vi "Data Display.vi"(8 "error in (no error)":errorcluster, 9 "UI Data Display Cluster":T3, 10 "Message Queues in":T1, 11 "Estimate Notifier in":refnum<notifier>) -> (0 "error out":errorcluster)   [LabVIEW 2019]
uses:
  controls/UI Display.ctl
  <vilib>/Math Plots/2D Math Plots/2D Compass/2D Compass XCtrl/2D Compass.xctl
  support/Message Queue/All Message Queues.ctl
  support/Message Queue/Message Cluster.ctl
  controls/Components Message Queues.ctl
  Data Analysis/EstimateCluster.ctl
  controls/Component Type.ctl
  support/Message Queue/Enqueue Message (Single).vi
  <vilib>/Math Plots/2D Math Plots/2D Compass/2D Compass Datatype/Public/Plot Helper (Vector).vi
  <vilib>/Utility/file.llb/Read Delimited Spreadsheet (DBL).vi
  <vilib>/Math Plots/2D Math Plots/2D Compass/2D Compass Datatype/Public/Plot Helper (Complex).vi
  <vilib>/Utility/error.llb/Error Cluster From Error Code.vi
  <vilib>/ErrorRing/Error Ring.xnode
  support/Message Queue/Message Queue.lvlib
  <vilib>/Math Plots/2D Math Plots/2D Compass/2D Compass Datatype/2D Compass Datatype.lvclass
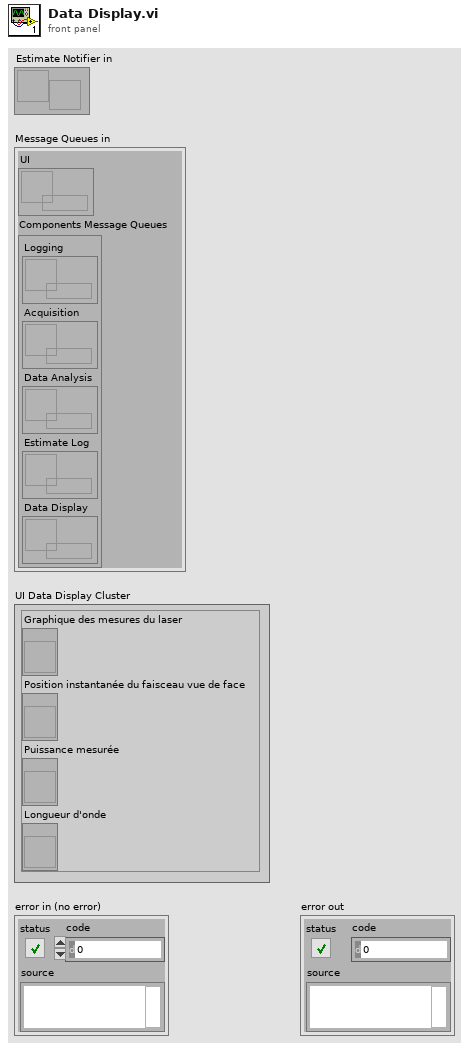
[diagram p1: front panel]
types:
  T1 = typedef "Message Queue.lvlib/All Message Queues.ctl" = cluster{"UI":refnum<queue>, "Components Message Queues":T2}
  T2 = typedef "Message Queue.lvlib/Components Message Queues.ctl" = cluster{"Logging":refnum<queue>, "Acquisition":refnum<queue>, "Data Analysis":refnum<queue>, "Estimate Log":refnum<queue>, "Data Display":refnum<queue>}
  T3 = typedef "UI Display.ctl" = cluster{"Graphique des mesures du laser":refnum<vi>, "Position instantanée du faisceau vue de face":refnum<vi>, "Puissance mesurée":refnum<vi>, "Longueur d'onde":refnum<vi>}
  T4 = typedef "Component Type.ctl" = enum16{"UI", "Logging", "Acquisition", "Data Analysis", "Estimate", "Data Display"}
  T5 = cluster{"all rows[0]":dbl, "all rows[1]":dbl, "all rows[2]":dbl, "all rows[3]":dbl, "all rows[4]":dbl, "all rows[5]":dbl, "all rows[6]":dbl, "all rows[7]":dbl, "all rows[8]":dbl}
  T6 = typedef "EstimateCluster.ctl" = cluster{"Lambda":dbl, "Puissance":dbl, "Rayon":dbl, "Angle":dbl, "dt":dbl, "t0":timestamp}
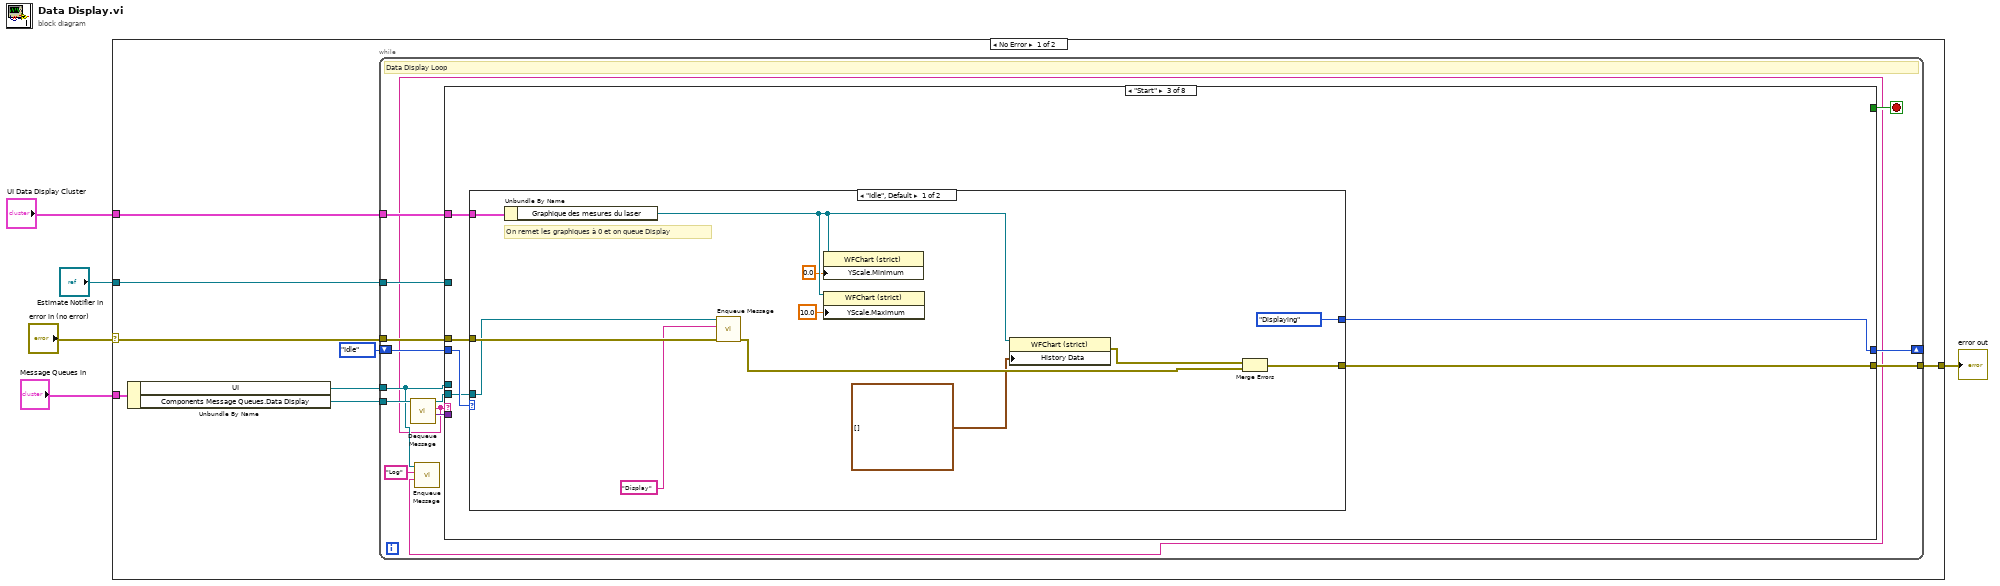
[diagram p0: block diagram]
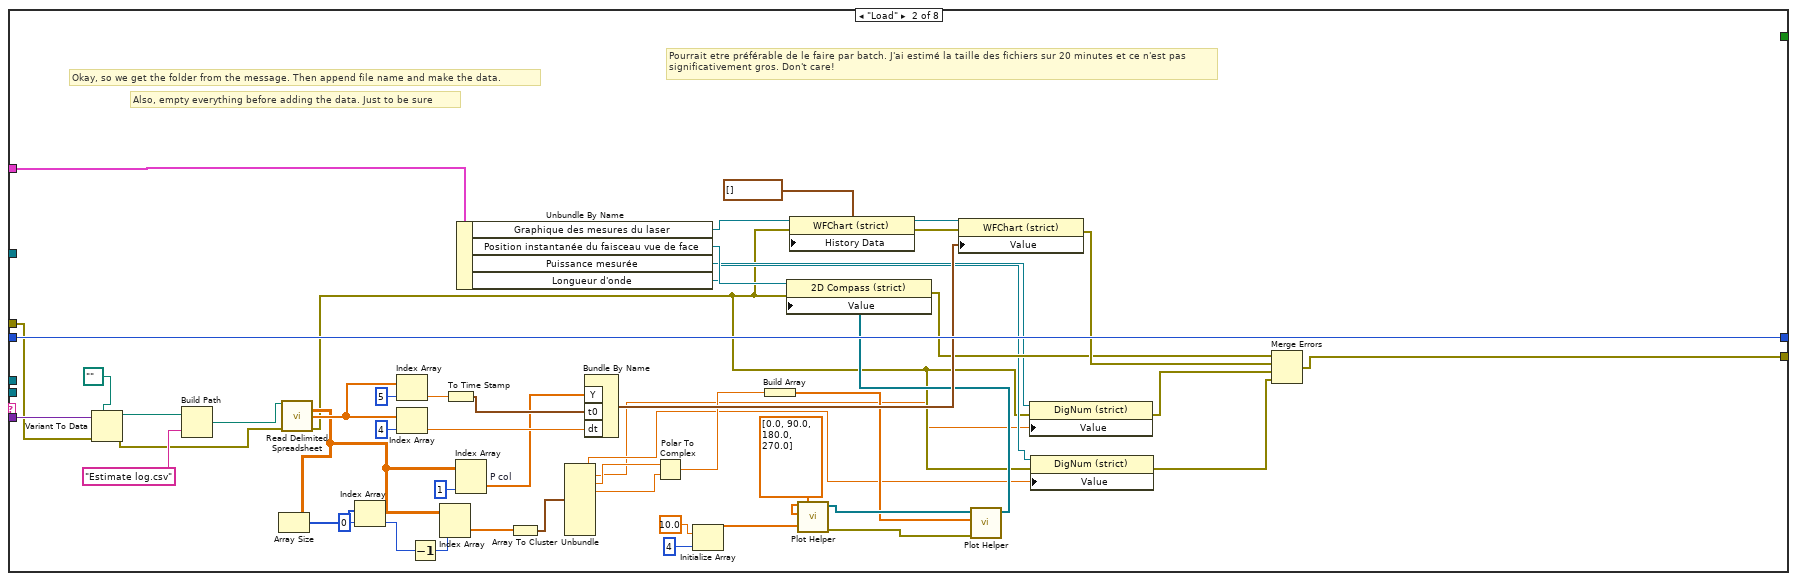
[diagram p3: hidden frame]
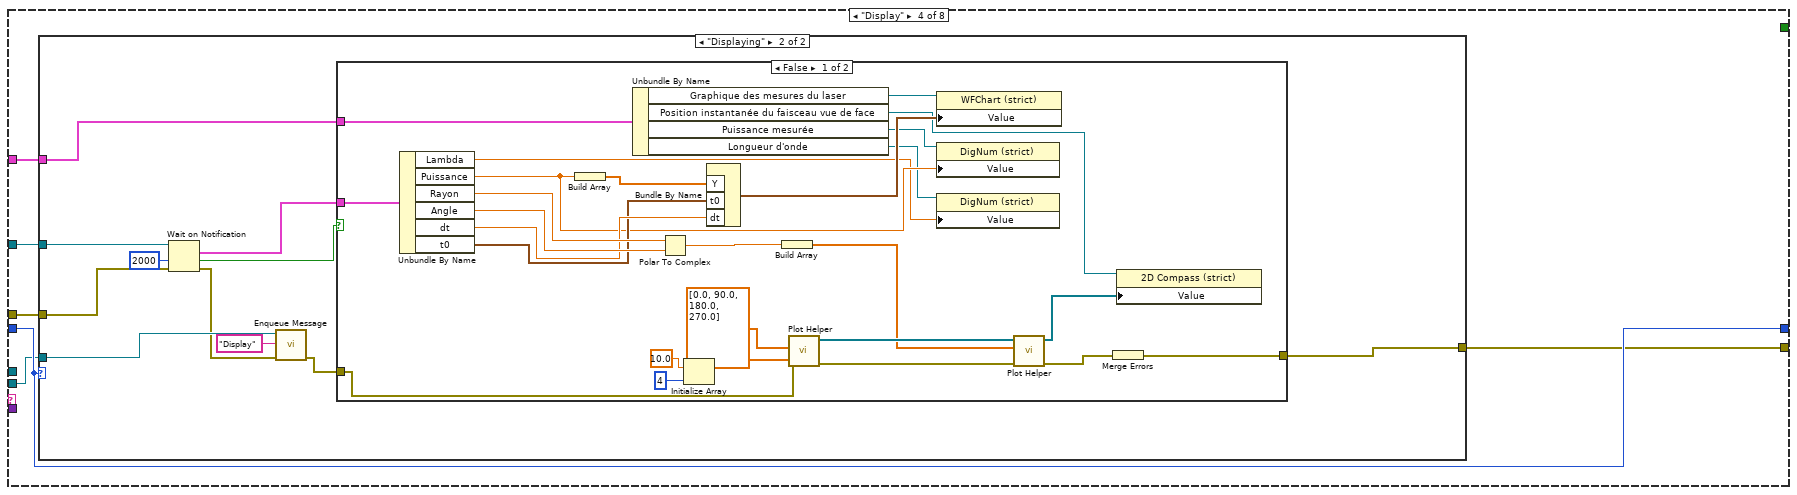
[diagram p5: hidden frame]
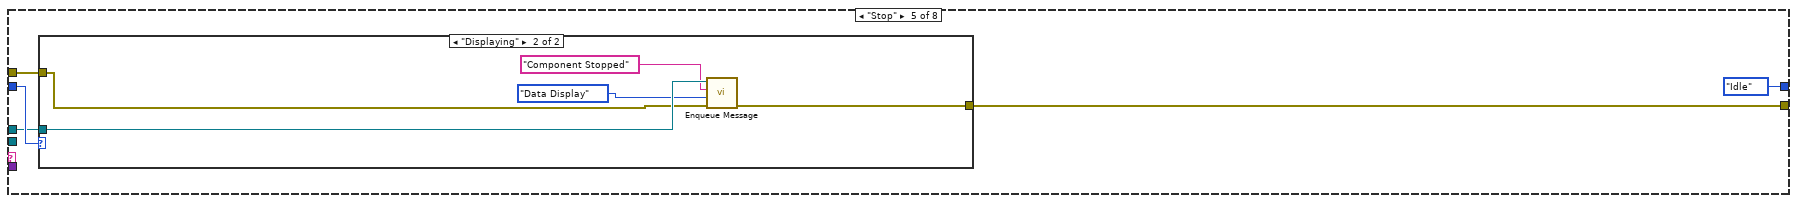
[diagram p8: hidden frame]
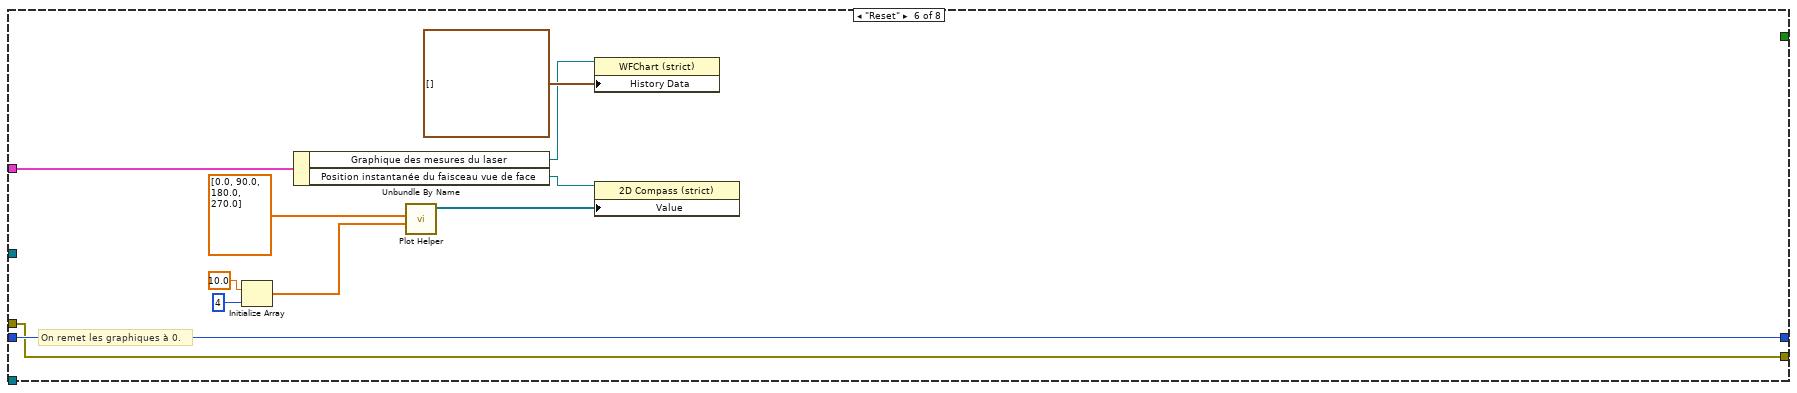
[diagram p10: hidden frame]
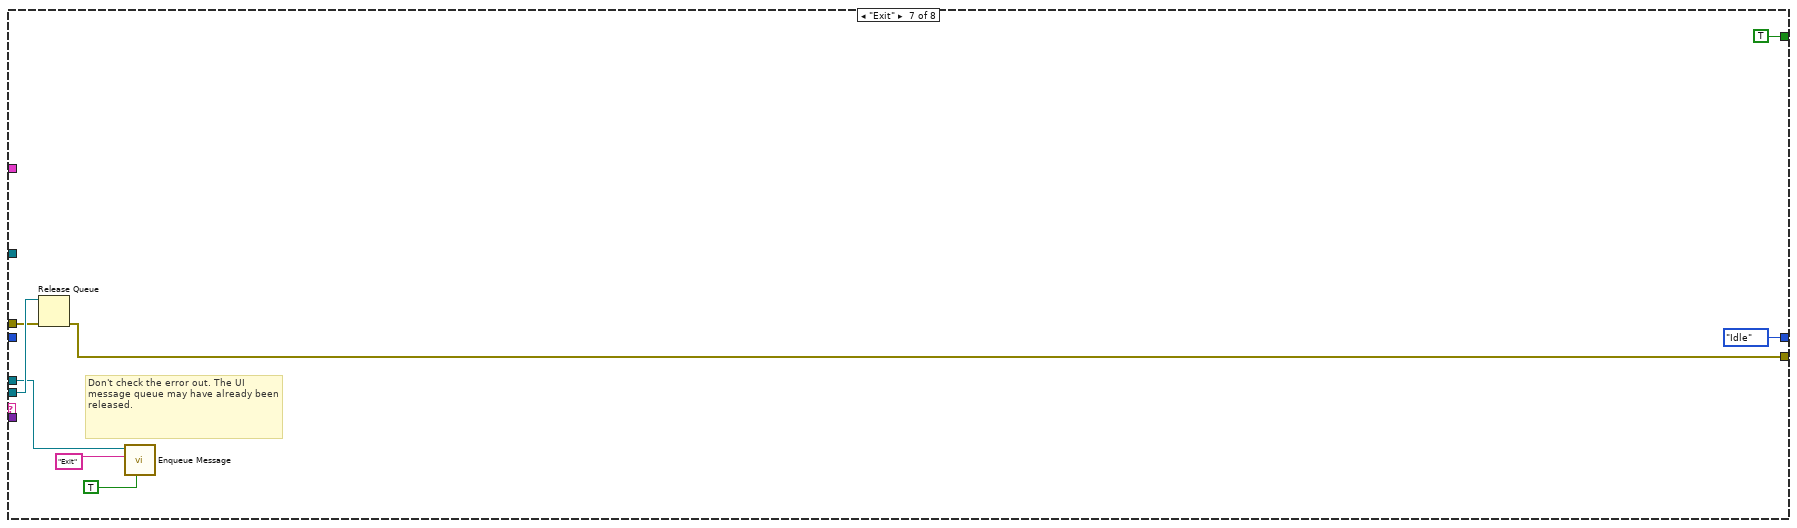
[diagram p11: hidden frame]
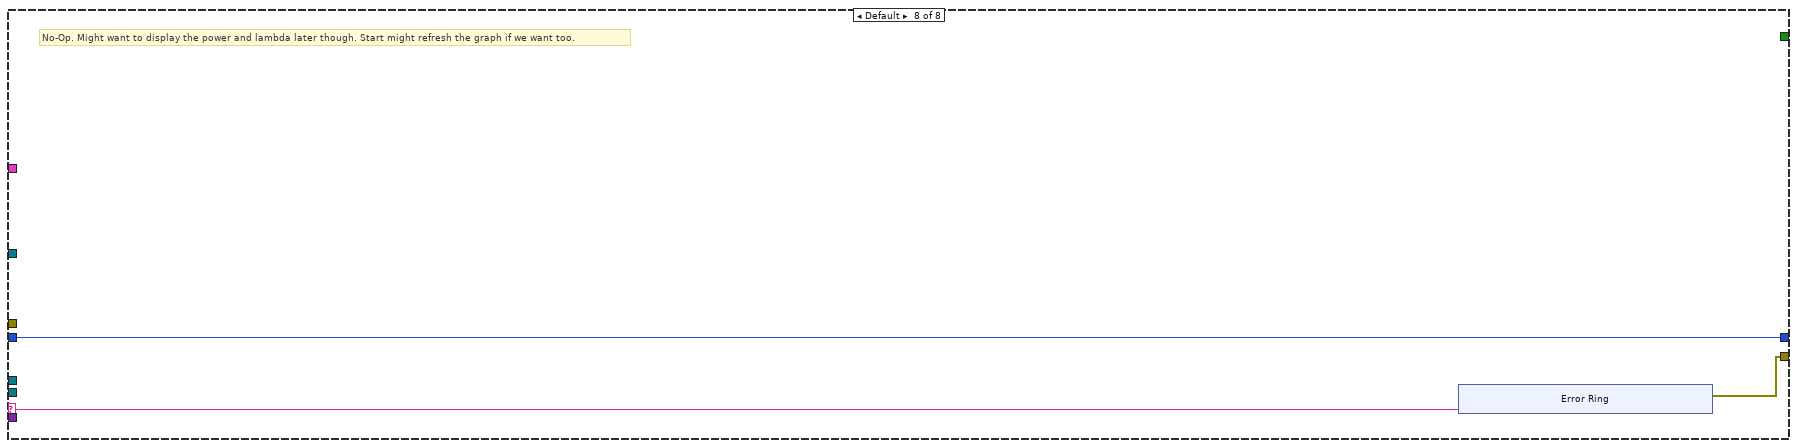
[diagram p12: hidden frame]
diagram:
  n1 = case shown="No Error" "error in (no error)" {
    selector: "error in (no error)" -> [w6 w185]
    tunnel: "Estimate Notifier in" -> [w13 _]
    tunnel: [w12 w185] -> w3
    tunnel: "Message Queues in" -> [w10 _]
    tunnel: "UI Data Display Cluster" -> [w7 _]
    frame No Error {
      n2 = Unbundle By Name(w10) -> ("UI"=w9:refnum<queue>, "Components Message Queues.Data Display"=w8:refnum<queue>)
      n3 = while "Data Display Loop" {
        tunnel: w13 -> [w25]
        tunnel: w8 -> [w26]
        tunnel: w6 -> [w23]
        tunnel: [w22] -> w12
        shift-right: [w20] -> _
        shift-left: enum16{"Idle", "Displaying"}."Idle" ("State") -> [w21]
        tunnel: w9 -> [w15]
        tunnel: w7 -> [w18]
        stop <- w24 stop-if-true
        # "Data Display Loop"
        n4 = call "Dequeue Message.vi"("Message Queue"=w26) -> ("Message Data"=w17:variant, "Message"=w14:string, "dup Message Queue"=w19:refnum<queue>)  [unwired: 7 in, 1 out]
        n5 = call-poly "Enqueue Message.vi"("Message Data"=w14, "Message"="Log", "Message Queue"=w15) -> ()  [unwired: 7 in, 2 out]
        n6 = case shown="\"Start\"" w14 {
          selector: w14 -> [_ _ _ _ _ _ _ w176]
          tunnel: w25 -> [_ _ _ w105 _ _ _ _]
          tunnel: [_ _ _ _ _ _ TRUE _] -> w24
          tunnel: w23 -> [w28 w29 w84 w102 w146 w165 w172 _]
          tunnel: [w28 w75 w83 w101 w145 w165 w171 w175] -> w22
          tunnel: w21 -> [w27 w79 w85 w104 w149 w166 _ w177]
          tunnel: [w27 w79 w82 w104 enum16{"Idle", "Displaying"}."Idle" ("State") w166 enum16{"Idle", "Displaying"}."Idle" ("State") w177] -> w20
          tunnel: w19 -> [_ _ w81 w103 _ _ w173 _]
          tunnel: w15 -> [_ _ _ _ w147 _ w168 _]
          tunnel: w18 -> [_ w67 w80 w100 _ w156 _ _]
          tunnel: w17 -> [_ w78 _ _ _ _ _ _]
          frame "Initialize" {
            # "No-Op. Might want to display the power and lambda later though. Start might refresh the graph if we want too."
          }
          frame "Load" {
            # "Pourrait etre préférable de le faire par batch. J'ai estimé la taille des fichiers sur 20 minutes et ce n'est pas\nsignificativement gros. Don't care!"
            # "Also, empty everything before adding the data. Just to be sure"
            # "Okay, so we get the folder from the message. Then append file name and make the data."
            n7 = Variant To Data(error in=w29, type=path "" ("base path"), Variant=w78) -> (data=w76:path, error out=w61:errorcluster)
            n8 = Build Path(base path=w76, name or relative path="Estimate log.csv") -> (appended path=w73:path)
            n9 = call-poly <vilib>:"Read Delimited Spreadsheet.vi"("file path (dialog if empty)"=w73, "error in (no error)"=w61) -> ("all rows"=w59:dbl[][], "first row"=w71:dbl[], "error out"=w40:errorcluster)  [unwired: 8 in, 3 out]
            n10 = Array Size(array=w59) -> (size(s)=w58:i32[])
            n11 = Index Array(array=w58, index=0) -> (element=w31:i32)
            n12 = Index Array(array=w71, index=5) -> (element=w70:dbl)
            n13 = Index Array(array=w71, index=4) -> (element=w72:dbl)
            n14 = Decrement(x=w31) -> (x-1=w30:i32)
            n15 = Index Array(array=w59, index (row)=w30) -> (element=w57:dbl[])  [unwired: 1 in]
            n16 = To Time Stamp(1:w70) -> (0:w69:timestamp)
            n17 = Index Array "P col"(array=w59, index (col)=1 ("disabled index (col)")) -> (element=w68:dbl[])  [unwired: 1 in]
            n18 = Unbundle By Name(w67) -> ("Graphique des mesures du laser"=w66:refnum<vi>, "Position instantanée du faisceau vue de face"=w55:refnum<vi>, "Puissance mesurée"=w42:refnum<vi>, "Longueur d'onde"=w41:refnum<vi>)
            n19 = Array To Cluster(array=w57) -> (cluster=w56:T5)
            n20 = Unbundle(w56) -> ("all rows[0]"=w39:dbl, "all rows[1]"=w38:dbl, "all rows[2]"=w45:dbl, "all rows[3]"=w44:dbl)  [unwired: 5 out]
            n21 = Bundle By Name("Y"=w68, "t0"=w69, "dt"=w72) -> (w63:waveform(dbl))  [unwired: 1 in]
            n22 = Polar To Complex(1:w44, 2:w45) -> (0:w50:cdb)
            n23 = Initialize Array(10.0 ("element"), 4 ("dimension size")) -> (w53:dbl[])
            n24 = Build Array(w50) -> (w49:cdb[])
            n25 = property class="WFChart (strict)"(reference=w66, error in=w40, "History Data"=waveform(dbl)[] []) -> (reference out=w65:refnum<vi>, error out=w62:errorcluster)
            n26 = call-poly <vilib>:"Plot Helper.vi"("radius vector"=w53, "theta vector"=dbl[] [0.0, 90.0, 180.0, 270.0]) -> ("error out"=w51:errorcluster, "2D Plot Class Obj Array out"=w52:refnum<class "2D Plot Datatype.lvclass">[])  [unwired: 2 in, 6 out]
            n27 = property class="WFChart (strict)"(reference=w65, error in=w62, "Value"=w63) -> (error out=w60:errorcluster)  [unwired: 1 out]
            n28 = call-poly <vilib>:"Plot Helper.vi"("error in (no error)"=w51, "z vector"=w49, "2D Plot Class Obj Array in"=w52) -> ("2D Plot Class Obj Array out"=w43:refnum<class "2D Plot Datatype.lvclass">[])  [unwired: 8 out]
            n29 = property class="2D Compass (strict)"(reference=w55, error in=w40, "Value"=w43) -> (error out=w54:errorcluster)  [unwired: 1 out]
            n30 = property class="DigNum (strict)"(reference=w42, error in=w40, "Value"=w38) -> (error out=w37:errorcluster)  [unwired: 1 out]
            n31 = property class="DigNum (strict)"(reference=w41, error in=w40, "Value"=w39) -> (error out=w36:errorcluster)  [unwired: 1 out]
            n32 = Merge Errors(w54, w60, w37, w36) -> (w75:errorcluster)
          }
          frame "Start" {
            n33 = case shown="\"Idle\", Default" w85 {
              selector: w85 -> [_ w98]
              tunnel: w84 -> [w96 w99]
              tunnel: [w93 w99] -> w83
              tunnel: [enum16{"Idle", "Displaying"}."Displaying" ("State") w98] -> w82
              tunnel: w81 -> [w91 _]
              tunnel: w80 -> [w89 _]
              frame "Idle", Default {
                # "On remet les graphiques à 0 et on queue Display"
                n34 = Unbundle By Name(w89) -> ("Graphique des mesures du laser"=w88:refnum<vi>)
                n35 = call-poly "Enqueue Message.vi"("error in (no error)"=w96, "Message"="Display", "Message Queue"=w91) -> ("error out"=w94:errorcluster)  [unwired: 7 in, 1 out]
                n36 = property class="WFChart (strict)"(reference=w88, "YScale.Minimum"=0.0 ("Y Scale.Range:Minimum")) -> ()  [unwired: 1 in, 2 out]
                n37 = property class="WFChart (strict)"(reference=w88, "YScale.Maximum"=10.0 ("Y Scale.Range:Maximum")) -> ()  [unwired: 1 in, 2 out]
                n38 = property class="WFChart (strict)"(reference=w88, "History Data"=waveform(dbl)[] []) -> (error out=w95:errorcluster)  [unwired: 1 in, 1 out]
                n39 = Merge Errors(w95, w94) -> (w93:errorcluster)
              }
              frame "Displaying" {
                # "Already running. Not sure why though"
              }
            }
          }
          frame "Display" {
            n40 = case shown="\"Displaying\"" w104 {
              tunnel: w105 -> [_ w116]
              tunnel: w103 -> [_ w115]
              tunnel: w102 -> [w106 w111]
              tunnel: [w106 w113] -> w101
              tunnel: w100 -> [_ w112]
              frame "Idle", Default {
                # "It has been stoped but the queue wasn't flushed out of Display message. Just ignore it. No op"
              }
              frame "Displaying" {
                n41 = Wait on Notification(notifier=w116, timeout in ms (-1)=2000, error in (no error)=w111) -> (notification=w117:T6, timed out?=w107:bool, error out=w110:errorcluster)  [unwired: 1 in, 1 out]
                n42 = call-poly "Enqueue Message.vi"("error in (no error)"=w110, "Message"="Display", "Message Queue"=w115) -> ("error out"=w109:errorcluster)  [unwired: 7 in, 1 out]
                n43 = case shown="False" w107 {
                  tunnel: w117 -> [w140 _]
                  tunnel: [w131 w144] -> w113
                  tunnel: w112 -> [w127 _]
                  tunnel: w109 -> [w118 w144]
                  frame False {
                    n44 = Unbundle By Name(w140) -> ("Lambda"=w119:dbl, "Puissance"=w121:dbl, "Rayon"=w138:dbl, "Angle"=w139:dbl, "dt"=w129:dbl, "t0"=w128:timestamp)
                    n45 = Build Array(w121) -> (w130:dbl[])
                    n46 = Unbundle By Name(w127) -> ("Graphique des mesures du laser"=w125:refnum<vi>, "Position instantanée du faisceau vue de face"=w123:refnum<vi>, "Puissance mesurée"=w122:refnum<vi>, "Longueur d'onde"=w120:refnum<vi>)
                    n47 = Polar To Complex(1:w139, 2:w138) -> (0:w137:cdb)
                    n48 = Initialize Array(10.0 ("element"), 4 ("dimension size")) -> (w143:dbl[])
                    n49 = Bundle By Name("Y"=w130, "t0"=w128, "dt"=w129) -> (w126:waveform(dbl))  [unwired: 1 in]
                    n50 = Build Array(w137) -> (w136:cdb[])
                    n51 = call-poly <vilib>:"Plot Helper.vi"("error in (no error)"=w118, "radius vector"=w143, "theta vector"=dbl[] [0.0, 90.0, 180.0, 270.0]) -> ("error out"=w141:errorcluster, "2D Plot Class Obj Array out"=w142:refnum<class "2D Plot Datatype.lvclass">[])  [unwired: 1 in, 6 out]
                    n52 = property class="WFChart (strict)"(reference=w125, "Value"=w126) -> ()  [unwired: 1 in, 2 out]
                    n53 = property class="DigNum (strict)"(reference=w122, "Value"=w121) -> ()  [unwired: 1 in, 2 out]
                    n54 = property class="DigNum (strict)"(reference=w120, "Value"=w119) -> ()  [unwired: 1 in, 2 out]
                    n55 = call-poly <vilib>:"Plot Helper.vi"("error in (no error)"=w141, "z vector"=w136, "2D Plot Class Obj Array in"=w142) -> ("error out"=w132:errorcluster, "2D Plot Class Obj Array out"=w124:refnum<class "2D Plot Datatype.lvclass">[])  [unwired: 7 out]
                    n56 = Merge Errors(w132) -> (w131:errorcluster)
                    n57 = property class="2D Compass (strict)"(reference=w123, "Value"=w124) -> ()  [unwired: 1 in, 2 out]
                  }
                  frame True {
                  }
                }
              }
            }
          }
          frame "Stop" {
            n58 = case shown="\"Displaying\"" w149 {
              tunnel: w147 -> [_ w155]
              tunnel: w146 -> [w150 w154]
              tunnel: [w150 w153] -> w145
              frame "Idle", Default {
              }
              frame "Displaying" {
                n59 = call-poly "Enqueue Message.vi"("error in (no error)"=w154, "Message Data"=Component_Type."Data Display" ("Component Type"), "Message"="Component Stopped", "Message Queue"=w155) -> ("error out"=w153:errorcluster)  [unwired: 6 in, 1 out]
              }
            }
          }
          frame "Reset" {
            # "On remet les graphiques à 0."
            n60 = Initialize Array(10.0 ("element"), 4 ("dimension size")) -> (w163:dbl[])
            n61 = Unbundle By Name(w156) -> ("Graphique des mesures du laser"=w157:refnum<vi>, "Position instantanée du faisceau vue de face"=w158:refnum<vi>)
            n62 = call-poly <vilib>:"Plot Helper.vi"("radius vector"=w163, "theta vector"=dbl[] [0.0, 90.0, 180.0, 270.0]) -> ("2D Plot Class Obj Array out"=w159:refnum<class "2D Plot Datatype.lvclass">[])  [unwired: 2 in, 7 out]
            n63 = property class="WFChart (strict)"(reference=w157, "History Data"=waveform(dbl)[] []) -> ()  [unwired: 1 in, 2 out]
            n64 = property class="2D Compass (strict)"(reference=w158, "Value"=w159) -> ()  [unwired: 1 in, 2 out]
          }
          frame "Exit" {
            # "Don't check the error out. The UI message queue may have already been released."
            n65 = Release Queue(queue=w173, error in (no error)=w172) -> (error out=w171:errorcluster)  [unwired: 1 in, 2 out]
            n66 = call-poly "Enqueue Message.vi"("Priority Message? (F)"=TRUE, "Message"="Exit", "Message Queue"=w168) -> ()  [unwired: 7 in, 2 out]
          }
          frame Default {
            # "No-Op. Might want to display the power and lambda later though. Start might refresh the graph if we want too."
            n67 = xnode "Error Ring"("parameter 0"=w176) -> ("error out"=w175:errorcluster)
          }
        }
      }
    }
    frame Error {
    }
  }
  "error out" <- w3
